vi "AFG1022 Test_2018.vi"() -> ()   [LabVIEW 2018]
doc: "Demonstrates how to configure then create an arbitrary waveform."
uses:
  C/Program Files (x86)/National Instruments/LabVIEW 2019/instr.lib/Tektronix AFG 1000 Series/Tektronix AFG 1000 Series.lvlib
panel:
  in  "Close Button":bool
  in  "Output Voltage, V":dbl(slide)=1.0 scale=-10.0..10.0 scale format="%#.2g"
  in  "Channel (1: Channel 1)":u16(ring)=1 items=["Channel 1"=1, "Channel 2"=2]
  in  "Enable Output":bool=TRUE
  in  "VISA resource name":refnum<visa-resource-name>
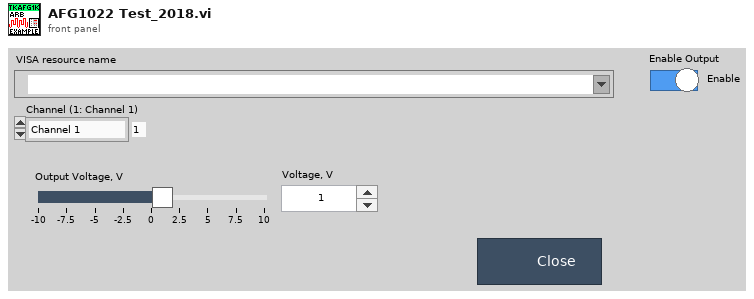
[diagram p1: front panel]
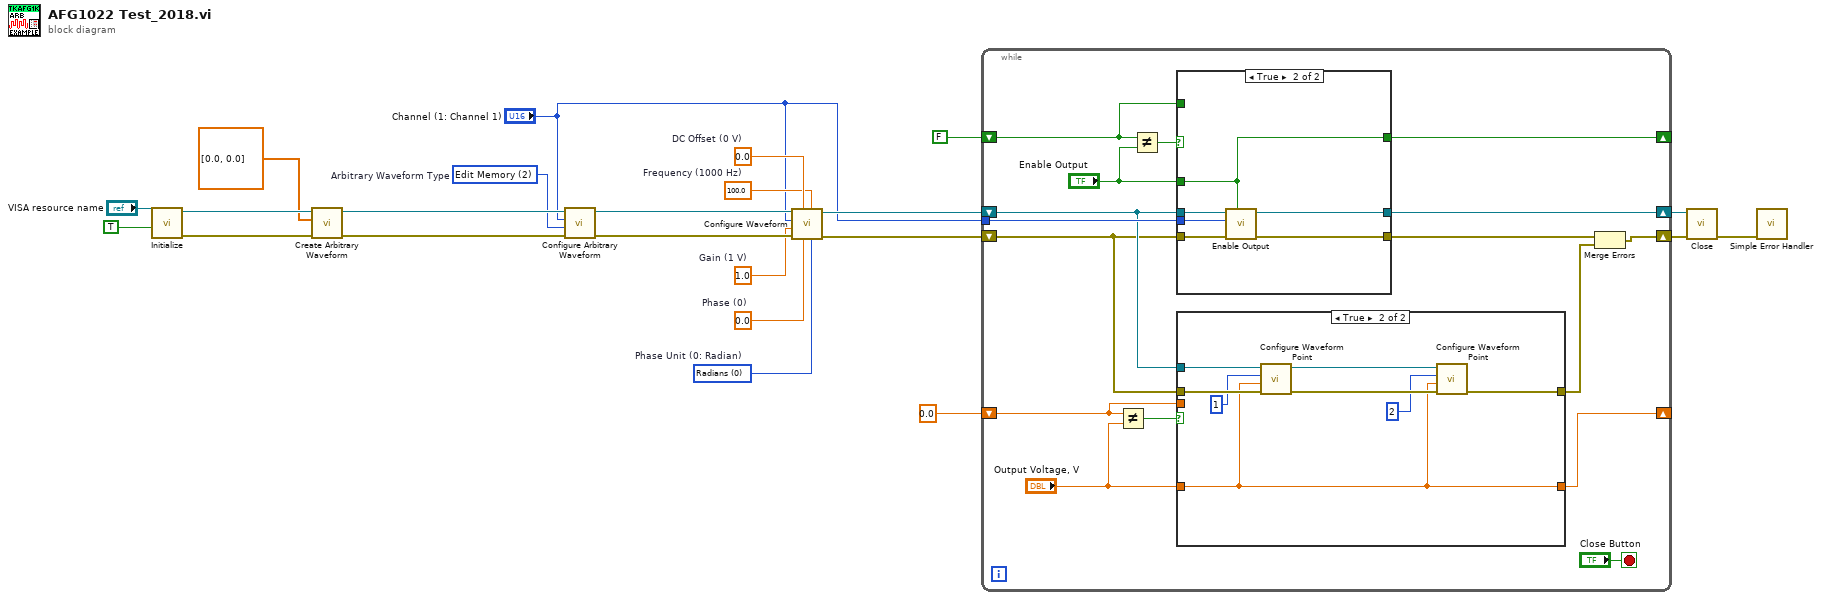
[diagram p0: block diagram]
diagram:
  w4 = 100.0  # Frequency (1000 Hz)
  w5 = 0.0  # DC Offset (0 V)
  w7 = u16 0 items=["Radians", "Degrees"]  # Phase Unit (0: Radian)
  w8 = 0.0  # Phase (0)
  w6 = 1.0  # Gain (1 V)
  w13 = u16 2 items=["Built-in", "User Waveform", "Edit Memory", "EFile"]  # Arbitrary Waveform Type
  n1 = call "Initialize.vi"("Reset (True)"=TRUE, "VISA resource name"="VISA resource name") -> ("error out"=w22:errorcluster, "VISA resource name out"=w20:refnum<visa-resource-name>)  [unwired: 8 in]
  n2 = call "Create Arbitrary Waveform.vi"("error in (no error)"=w22, "Arbitrary Waveform Data"=dbl[] [0.0, 0.0], "VISA resource name"=w20) -> ("error out"=w16:errorcluster, "VISA resource name out"=w17:refnum<visa-resource-name>)  [unwired: 7 in]
  n3 = call "Configure Arbitrary Waveform.vi"("error in (no error)"=w16, "Arbitrary Waveform Type (0: Built-in)"=w13, "Channel (1: Channel 1)"="Channel (1: Channel 1)", "VISA resource name"=w17) -> ("error out"=w12:errorcluster, "VISA resource name out"=w10:refnum<visa-resource-name>)  [unwired: 6 in]
  n4 = call "Configure Waveform.vi"("Phase Unit (0: Radian)"=w7, "Frequency (1000 Hz)"=w4, "Phase (0)"=w8, "DC Offset (0.00 V)"=w5, "error in (no error)"=w12, "Amplitude (1 Vpp)"=w6, "Channel (1 Channel 1)"="Channel (1: Channel 1)", "VISA resource name"=w10) -> ("error out"=w11:errorcluster, "VISA resource name out"=w9:refnum<visa-resource-name>)  [unwired: 2 in]
  n5 = while {
    tunnel: "Channel (1: Channel 1)" -> [w38]
    shift-right: [w29] -> w14
    shift-left: w11 -> [w30]
    shift-right: [w39] -> w15
    shift-left: w9 -> [w32]
    shift-right: [w26] -> _
    shift-left: 0.0 -> [w25]
    shift-right: [w35] -> _
    shift-left: FALSE -> [w34]
    stop <- "Close Button" stop-if-true
    n6 = Not Equal?(x=w25, y="Output Voltage, V") -> (x != y?=w33:bool)
    n7 = Not Equal?(x=w34, y="Enable Output") -> (x != y?=w37:bool)
    n8 = case shown="True" w37 {
      tunnel: [w52 w58] -> w39
      tunnel: [w51 w57] -> w28
      tunnel: w30 -> [w51 w56]
      tunnel: w32 -> [w52 w55]
      tunnel: w38 -> [_ w54]
      tunnel: "Enable Output" -> [_ w53]
      tunnel: [w50 w53] -> w35
      tunnel: w34 -> [w50 _]
      frame False {
      }
      frame True {
        n9 = call "Enable Output.vi"("Enable Output (T: Enable)"=w53, "error in (no error)"=w56, "Channel (1: Channel 1)"=w54, "VISA resource name"=w55) -> ("error out"=w57:errorcluster, "VISA resource name out"=w58:refnum<visa-resource-name>)  [unwired: 6 in]
      }
    }
    n10 = case shown="True" w33 {
      tunnel: w32 -> [_ w49]
      tunnel: "Output Voltage, V" -> [_ w43]
      tunnel: w30 -> [w41 w48]
      tunnel: [w41 w45] -> w27
      tunnel: [w40 w43] -> w26
      tunnel: w25 -> [w40 _]
      frame False {
      }
      frame True {
        n11 = call "Configure Waveform Point.vi"("error in (no error)"=w48, "Value (1)"=w43, "Index (1)"=1, "VISA resource name"=w49) -> ("error out"=w46:errorcluster, "VISA resource name out"=w44:refnum<visa-resource-name>)  [unwired: 6 in]
        n12 = call "Configure Waveform Point.vi"("error in (no error)"=w46, "Value (1)"=w43, "Index (1)"=2, "VISA resource name"=w44) -> ("error out"=w45:errorcluster)  [unwired: 6 in, 1 out]
      }
    }
    n13 = Merge Errors(w28, w27) -> (w29:errorcluster)
  }
  n14 = call "Close.vi"("error in (no error)"=w14, "VISA resource name"=w15) -> ("error out"=w23:errorcluster)  [unwired: 9 in]
  n15 = call <vilib>:"Simple Error Handler.vi"("error in (no error)"=w23) -> ()  [unwired: 4 in, 5 out]
